vi "CRYLoad Graph Main.vi"(4 "nData":i32, 5 "sAction":string, 6 "sQueue Name":string, 7 "Graph Main Ref":refnum<vi>, 8 "Spliter Ref Array":refnum<vi>[](array[refnum]), 9 "Panel Ref Array":refnum<vi>[](array[refnum]), 10 "DataView Index":i32, 11 "Flattend Data":string) -> (3 "Title State":bool)   [LabVIEW 2013]
uses:
  CRYNew View Global.vi
  CRYView Global.vi
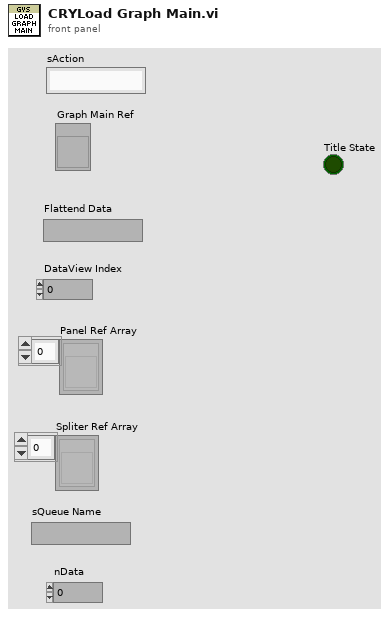
[diagram p1: front panel]
types:
  T1 = typedef "Graph Main Info Cluster.ctl" = cluster{"Selected_BarIdx":i32, "Selected_PanelIdx":i32, "Graph Main VIRef":refnum<vi>, "ToolBarClick":bool, "Spliter Ref Array":refnum<vi>[], "Panel Ref Array":refnum<vi>[], "Spliter_matrix":i32[][], "Panel_matrix":i32[][], "child_spliterIdx_matrix":i32[][], "split_pos_matrix":i32[][], "Title State":bool, "sQueueName":string, "Frame nID":i32, "Graph VIRef Array":cluster{"Graph VIRef":refnum<vi>, "Panel Idx":i32, "Frame VIRef":refnum<vi>, "Icon Ring":i32, "Graph Type":string}[], "View Type":string}
  T2 = cluster{"Graph VIRef":refnum<vi>, "Panel Idx":i32, "Frame VIRef":refnum<vi>, "Icon Ring":i32, "Graph Type":string}[]
  T3 = cluster{"sAction":string, "sData":string, "nData":i32, "pVIRef":refnum<vi>}
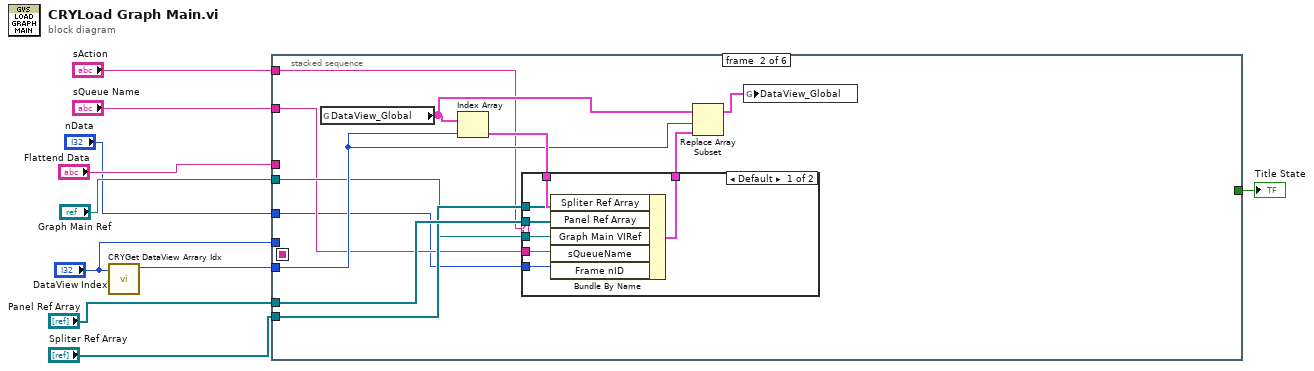
[diagram p0: block diagram]
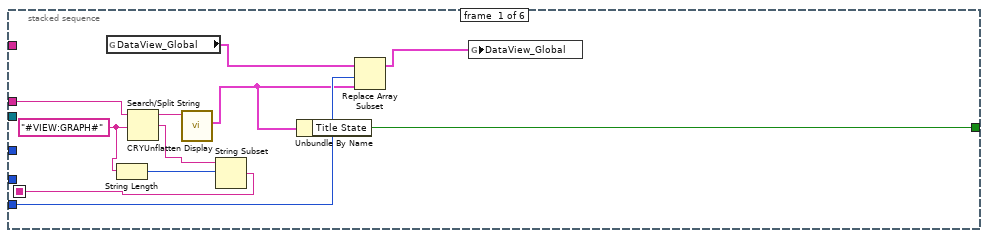
[diagram p2: hidden frame]
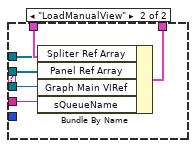
[diagram p3: hidden frame]
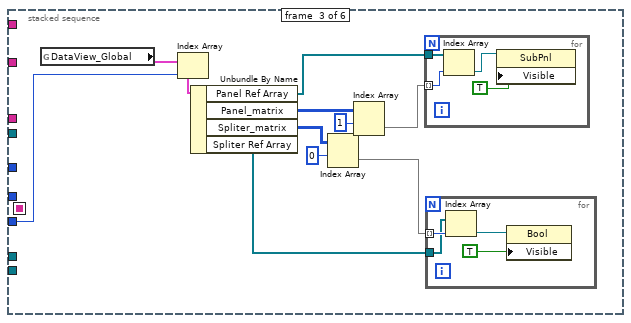
[diagram p4: hidden frame]
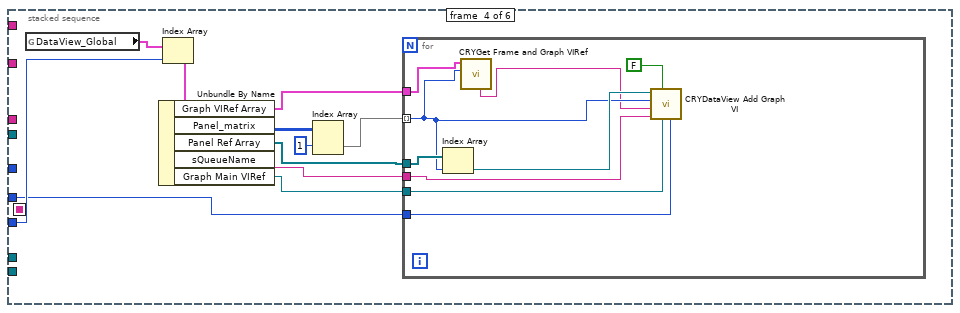
[diagram p5: hidden frame]
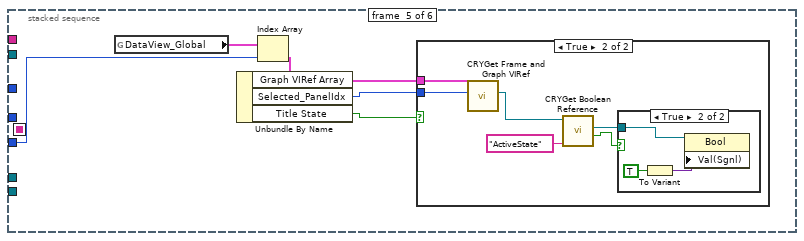
[diagram p6: hidden frame]
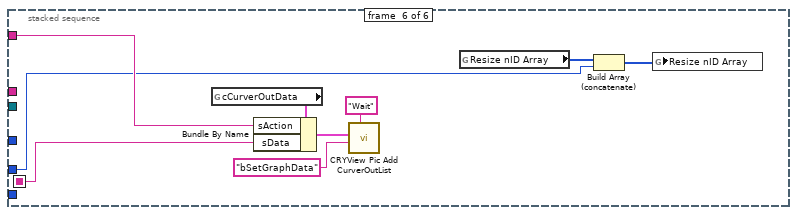
[diagram p9: hidden frame]
diagram:
  n1 = call "CRYGet DataView Arrary Idx.vi"("DataView Idx In"="DataView Index") -> ("DataView Arrary Idx out"=w9:i32)  [unwired: 10 in]
  n2 = stacked-sequence {
    seq-local: [w11 _ _ _ _ _] -> [_ _ _ _ _ w104]
    tunnel: "Flattend Data" -> [w20 _ _ _ _ _]
    tunnel: w9 -> [w17 w26 w46 w74 w87 _]
    tunnel: "Panel Ref Array" -> [_ w28 _ _ _ _]
    tunnel: "Spliter Ref Array" -> [_ w27 _ _ _ _]
    tunnel: "DataView Index" -> [_ _ _ w65 _ w101]
    tunnel: "Graph Main Ref" -> [_ w25 _ _ _ _]
    tunnel: "sQueue Name" -> [_ w24 _ _ _ w103]
    tunnel: "nData" -> [_ w23 _ _ _ _]
    tunnel: [w15 _ _ _ _ _] -> w2
    tunnel: "sAction" -> [_ w22 _ _ _ _]
    frame #0 {
      w13 = "#VIEW:GRAPH#" ("regular expression")
      n3 = global read "CRYNew View Global.vi" "DataView_Global"() -> (w19:T1[])
      n4 = String Length(string=w13) -> (length=w12:i32)
      n5 = Search/Split String(string=w20, search string/char (-)=w13) -> (substring before match=w21:string, match + rest of string=w14:string)  [unwired: 1 in, 1 out]
      n6 = call "CRYUnflatten Display.vi"("Flatten Display"=w21) -> ("DataView GUI Info"=w16:T1)  [unwired: 8 in, 2 out]
      n7 = String Subset(string=w14, offset (0)=w12) -> (substring=w11:string)  [unwired: 1 in]
      n8 = Unbundle By Name(w16) -> ("Title State"=w15:bool)
      n9 = Replace Array Subset(array=w19, new element=w16, index=w17) -> (w18:T1[])
      n10 = global write "CRYNew View Global.vi" "DataView_Global"(w18) -> ()
    }
    frame #1 {
      n11 = global read "CRYNew View Global.vi" "DataView_Global"() -> (w30:T1[])
      n12 = Index Array(array=w30, index=w26) -> (element=w32:T1)
      n13 = case shown="Default" w22 {
        tunnel: w32 -> [w39 w45]
        tunnel: [w38 w44] -> w29
        tunnel: w28 -> [w37 w43]
        tunnel: w27 -> [w36 w42]
        tunnel: w25 -> [w35 w41]
        tunnel: w24 -> [w34 w40]
        tunnel: w23 -> [w33 _]
        frame Default {
          n14 = Bundle By Name(cluster=w39, "Spliter Ref Array"=w36, "Panel Ref Array"=w37, "Graph Main VIRef"=w35, "sQueueName"=w34, "Frame nID"=w33) -> (w38:T1)
        }
        frame "LoadManualView" {
          n15 = Bundle By Name(cluster=w45, "Spliter Ref Array"=w42, "Panel Ref Array"=w43, "Graph Main VIRef"=w41, "sQueueName"=w40) -> (w44:T1)
        }
      }
      n16 = Replace Array Subset(array=w30, new element=w29, index=w26) -> (w31:T1[])
      n17 = global write "CRYNew View Global.vi" "DataView_Global"(w31) -> ()
    }
    frame #2 {
      n18 = global read "CRYNew View Global.vi" "DataView_Global"() -> (w56:T1[])
      n19 = Index Array(array=w56, index=w46) -> (element=w55:T1)
      n20 = Unbundle By Name(w55) -> ("Panel Ref Array"=w48:refnum<vi>[], "Panel_matrix"=w54:i32[][], "Spliter_matrix"=w51:i32[][], "Spliter Ref Array"=w47:refnum<vi>[])
      n21 = Index Array(array=w51, index (row)=0) -> (element=w50:i32[])  [unwired: 1 in]
      n22 = Index Array(array=w54, index (row)=1) -> (element=w49:i32[])  [unwired: 1 in]
      n23 = for {
        tunnel: w48 -> [w64]
        tunnel: w49 -> [w63] mode=indexing
        n24 = Index Array(array=w64, index=w63) -> (element=w62:refnum<vi>)
        n25 = property class="SubPnl"(reference=w62, "Visible"=TRUE) -> ()  [unwired: 1 in, 2 out]
      }
      n26 = for {
        tunnel: w47 -> [w59]
        tunnel: w50 -> [w60] mode=indexing
        n27 = Index Array(array=w59, index=w60) -> (element=w58:refnum<vi>)
        n28 = property class="Bool"(reference=w58, "Visible"=TRUE) -> ()  [unwired: 1 in, 2 out]
      }
    }
    frame #3 {
      n29 = global read "CRYNew View Global.vi" "DataView_Global"() -> (w75:T1[])
      n30 = Index Array(array=w75, index=w74) -> (element=w73:T1)
      n31 = Unbundle By Name(w73) -> ("Graph VIRef Array"=w69:T2, "Panel_matrix"=w72:i32[][], "Panel Ref Array"=w68:refnum<vi>[], "sQueueName"=w67:string, "Graph Main VIRef"=w66:refnum<vi>)
      n32 = Index Array(array=w72, index (row)=1) -> (element=w70:i32[])  [unwired: 1 in]
      n33 = for {
        tunnel: w70 -> [w77] mode=indexing
        tunnel: w69 -> [w78]
        tunnel: w68 -> [w84]
        tunnel: w67 -> [w82]
        tunnel: w66 -> [w81]
        tunnel: w65 -> [w80]
        n34 = Index Array(array=w84, index=w77) -> (element=w83:refnum<vi>)
        n35 = call "CRYGet Frame and Graph VIRef.vi"("Panel Idx"=w77, "Graph VIRef Array"=w78) -> ("Graph Type"=w76:string)  [unwired: 5 in, 4 out]
        n36 = call "CRYDataView Add Graph VI.vi"("DataView Idx"=w80, "Graph Main VIRef In"=w81, "isFirstPanel"=FALSE, "Queue Name"=w82, "GraphType"=w76, "panel_index"=w77, "Panel Ref In"=w83) -> ()  [unwired: 4 in, 1 out]
      }
    }
    frame #4 {
      n37 = global read "CRYNew View Global.vi" "DataView_Global"() -> (w86:T1[])
      n38 = Index Array(array=w86, index=w87) -> (element=w88:T1)
      n39 = Unbundle By Name(w88) -> ("Graph VIRef Array"=w89:T2, "Selected_PanelIdx"=w90:i32, "Title State"=w85:bool)
      n40 = case shown="True" w85 {
        tunnel: w90 -> [_ w94]
        tunnel: w89 -> [_ w93]
        frame False {
        }
        frame True {
          n41 = call "CRYGet Frame and Graph VIRef.vi"("Panel Idx"=w94, "Graph VIRef Array"=w93) -> ("Frame VIRef"=w95:refnum<vi>)  [unwired: 5 in, 4 out]
          n42 = call "CRYGet Boolean Reference.vi"("Label Name"="ActiveState", "VI Refnum"=w95) -> ("Exist?"=w91:bool, "Boolean Ref"=w92:refnum<vi>)  [unwired: 7 in, 1 out]
          n43 = case shown="True" w91 {
            tunnel: w92 -> [_ w97]
            frame False {
            }
            frame True {
              n44 = To Variant(anything=TRUE) -> (Variant=w99:variant)
              n45 = property class="Bool"(reference=w97, "Val(Sgnl)"=w99) -> ()  [unwired: 1 in, 2 out]
            }
          }
        }
      }
    }
    frame #5 {
      n46 = global read "CRYView Global.vi" "cCurverOutData"() -> (w108:T3)
      n47 = Bundle By Name(cluster=w108, "sAction"=w103, "sData"=w104) -> (w105:T3)
      n48 = call "CRYView Pic Add CurverOutList.vi"("sAction"="Wait", "sName"="bSetGraphData" ("Label Name"), "cCurverOutData"=w105) -> ()  [unwired: 9 in]
      n49 = global read "CRYNew View Global.vi" "Resize nID Array"() -> (w102:i32[])
      n50 = Build Array (concatenate)(w102, w101) -> (w100:i32[])
      n51 = global write "CRYNew View Global.vi" "Resize nID Array"(w100) -> ()
    }
  }
  "Title State" <- w2
